vi "DisplayErrorsForDevice.vi"(0 "CmdLib In":refnum<k24>, 1 "Device Key":string, 2 "Device Address":i32, 3 "Prefix":string, 4 "Status:":refnum<vi>, 5 "error in":errorcluster) -> (14 "CmdLib Out":refnum<k24>, 15 "DeviceKey Out":string, 16 "Device Address Out":i32, 19 "error out":errorcluster)   [LabVIEW 2012]
uses:
  D:/workspace/GitHub/LVsolis/lib/CmdLib.dll
  lib/CmdLib.dll
  <vilib>/regexp/Match Regular Expression.xnode
panel:
  in  "errMsg":string
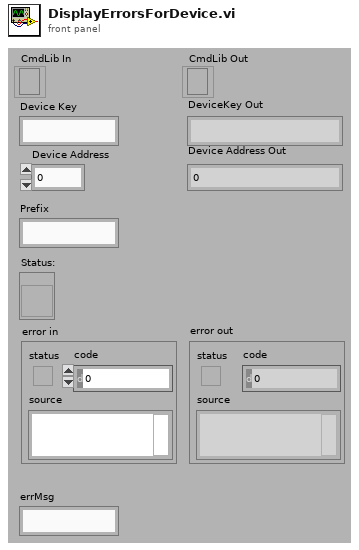
[diagram p1: front panel]
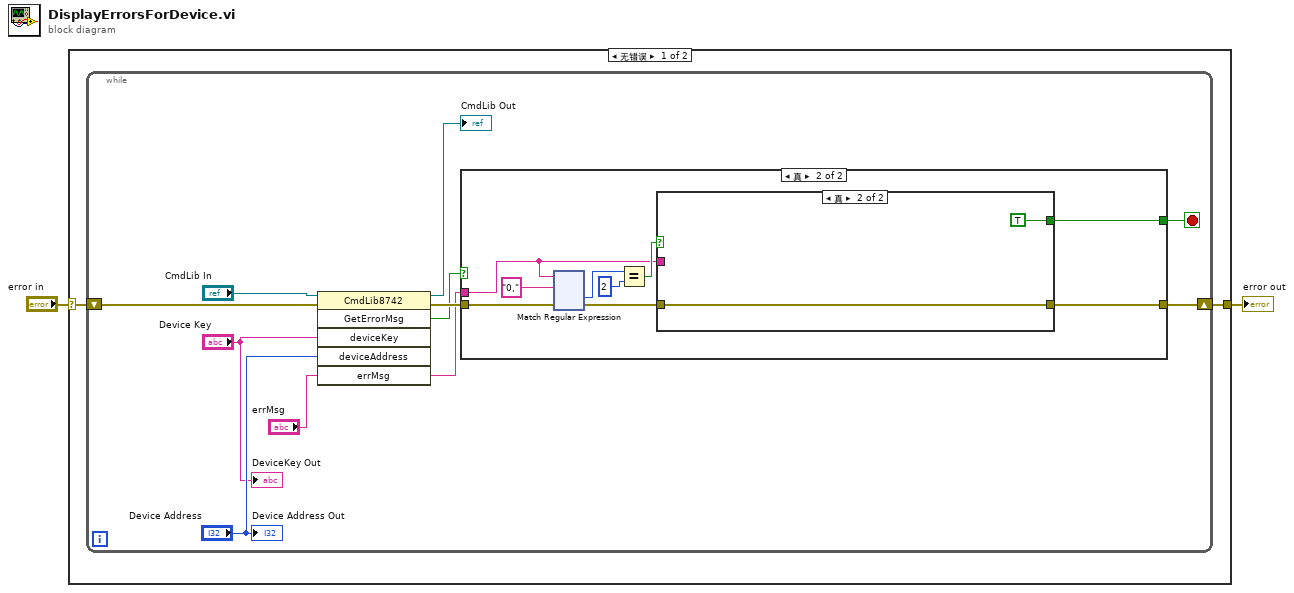
[diagram p0: block diagram]
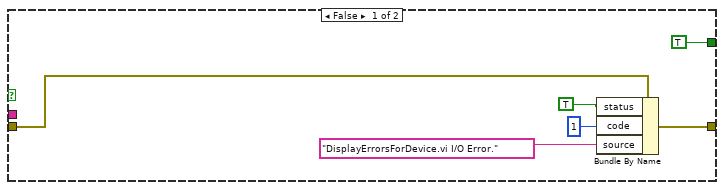
[diagram p2: hidden frame]
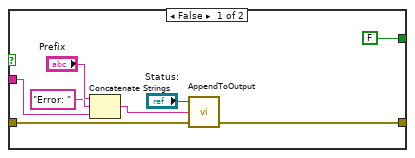
[diagram p3: hidden frame]
diagram:
  n1 = case shown="无错误" "error in" {
    selector: "error in" -> [w4 w152]
    tunnel: [w3 w152] -> w1
    frame No Error {
      n2 = while {
        shift-right: [w12] -> w3
        shift-left: w4 -> [w13]
        stop <- w5 stop-if-true
        n3 = invoke class="CmdLib8742" method="GetErrorMsg"(reference="CmdLib In", error in=w13, "deviceKey"="Device Key", "deviceAddress"="Device Address", "errMsg"="errMsg") -> (reference out=→"CmdLib Out":refnum<k24>, error out=w14:errorcluster, "GetErrorMsg"=w6:bool, "errMsg"=w7:string)  [unwired: 1 in, 2 out]
        n4 = case shown="真" w6 {
          tunnel: w14 -> [w21 w24]
          tunnel: [w16 w27] -> w12
          tunnel: w7 -> [_ w22]
          tunnel: [TRUE w28] -> w5
          frame False {
            n5 = Bundle By Name(cluster=w21, "status"=TRUE, "code"=1, "source"="DisplayErrorsForDevice.vi I/O Error.") -> (w16:errorcluster)
          }
          frame True {
            n6 = xnode "Match Regular Expression"("输入字符串"=w22, "正则表达式"="0," ("regular expression"), "错误输入"=w24) -> ("匹配后偏移量"=w26:i32, "错误输出"=w25:errorcluster)  [unwired: 3 in, 3 out]
            n7 = Equal?(x=w26, y=2) -> (x = y?=w29:bool)
            n8 = case shown="真" w29 {
              tunnel: [FALSE TRUE] -> w28
              tunnel: w25 -> [w144 w150]
              tunnel: w22 -> [w143 _]
              tunnel: [w142 w150] -> w27
              frame False {
                n9 = Concatenate Strings("Prefix", "Error: ", w143) -> (w149:string)
                n10 = call "AppendToOutput.vi"("error in"=w144, "Input String"=w149, "Output Refnum In"="Status:") -> ("error out"=w142:errorcluster)  [unwired: 1 in, 1 out]
              }
              frame True {
              }
            }
          }
        }
        "DeviceKey Out" <- "Device Key"
        "Device Address Out" <- "Device Address"
      }
    }
    frame Error {
    }
  }
  "error out" <- w1
